vi "On Off.vi"(8 "error in (no error)":errorcluster, 10 "On Off":bool, 11 "State in":refnum<class "Parent Actor.lvclass">) -> (0 "error out":errorcluster, 3 "State out":refnum<class "Parent Actor.lvclass">)   [LabVIEW 2015, in "Parent Actor.lvclass"]
uses:
  Parent Actor.lvclass
  Parent Actor.lvclass/Parent Actor.ctl
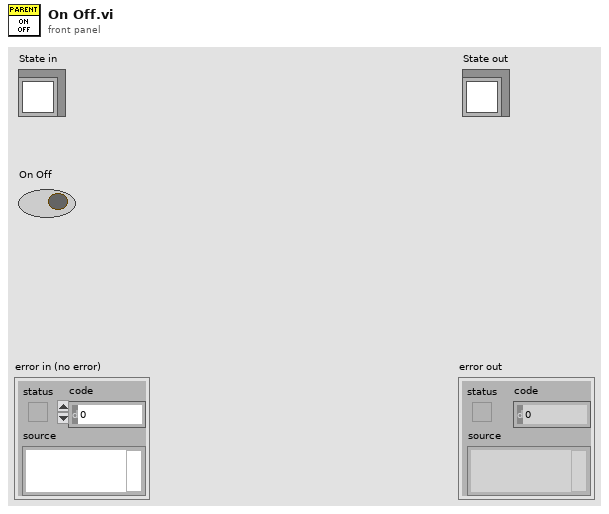
[diagram p1: front panel]
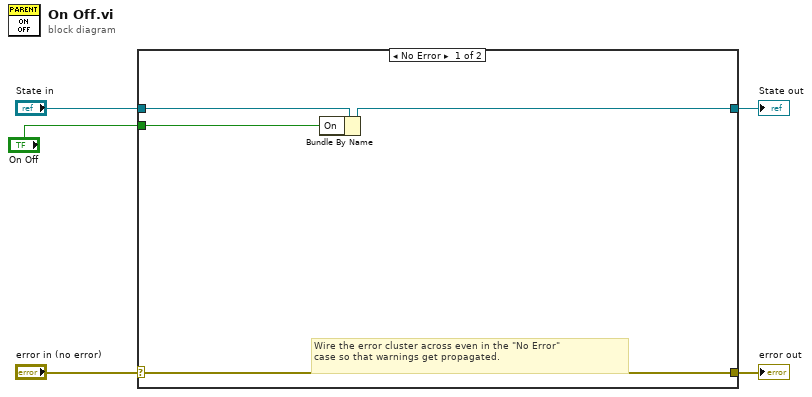
[diagram p0: block diagram]
diagram:
  n1 = case shown="No Error" "error in (no error)" {
    selector: "error in (no error)" -> [w8 w11]
    tunnel: [w8 w11] -> w4
    tunnel: [w7 w10] -> w2
    tunnel: "State in" -> [w9 w10]
    tunnel: "On Off" -> [w6 _]
    frame No Error {
      # "Wire the error cluster across even in the \"No Error\"\ncase so that warnings get propagated."
      n2 = Bundle By Name(cluster=w9, "On"=w6) -> (w7:refnum<class "Parent Actor.lvclass">)
    }
    frame Error {
    }
  }
  "error out" <- w4
  "State out" <- w2
